vi "GVSGet Boolean Reference.vi"(8 "Label Name":string, 11 "VI Refnum":refnum<vi>) -> (1 "Boolean":bool, 2 "Boolean Ref":refnum<vi>, 3 "VI Refnum Out":refnum<vi>)   [LabVIEW 2013]
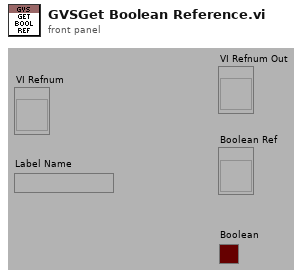
[diagram p1: front panel]
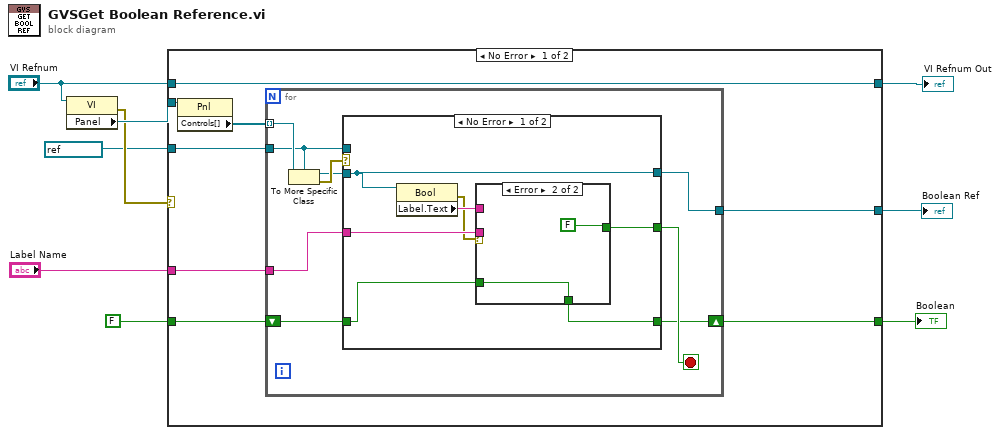
[diagram p0: block diagram]
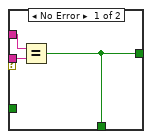
[diagram p2: hidden frame]
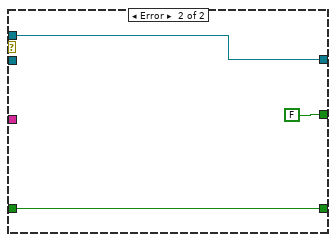
[diagram p3: hidden frame]
diagram:
  n1 = property class="VI"(reference="VI Refnum") -> (error out=w6:errorcluster, "Panel"=w8:refnum<vi>)  [unwired: 1 in, 1 out]
  n2 = case shown="No Error" w6 {
    tunnel: "Label Name" -> [w17 _]
    tunnel: w8 -> [w16 _]
    tunnel: "VI Refnum" -> [w11 w44]
    tunnel: FALSE ("Boolean") -> [w14 w42]
    tunnel: [w13 w42] -> w4
    tunnel: [w12 w43] -> w3
    tunnel: [w11 w44] -> w2
    tunnel: refnum<vi> refnum ("Boolean") -> [w10 w43]
    frame No Error {
      n3 = property class="Pnl"(reference=w16) -> ("Controls[]"=w15:refnum<vi>[])  [unwired: 1 in, 2 out]
      n4 = for {
        tunnel: w15 -> [w26] mode=indexing
        tunnel: [w22] -> w12
        tunnel: w17 -> [w21]
        tunnel: w10 -> [w20]
        shift-right: [w18] -> w13
        shift-left: w14 -> [w19]
        stop <- w23 stop-if-true
        n5 = To More Specific Class(target class=w20, reference=w26) -> (specific class reference=w24:refnum<vi>, error out=w25:errorcluster)  [unwired: 1 in]
        n6 = case shown="No Error" w25 {
          tunnel: w24 -> [w31 _]
          tunnel: [w29 FALSE] -> w23
          tunnel: [w31 w40] -> w22
          tunnel: w21 -> [w32 _]
          tunnel: w20 -> [_ w40]
          tunnel: [w28 w39] -> w18
          tunnel: w19 -> [w27 w39]
          frame No Error {
            n7 = property class="Bool"(reference=w31) -> (error out=w30:errorcluster, "Label.Text"=w33:string)  [unwired: 1 in, 1 out]
            n8 = case shown="Error" w30 {
              tunnel: w33 -> [w36 _]
              tunnel: w32 -> [w35 _]
              tunnel: [w34 FALSE] -> w29
              tunnel: [w34 w37] -> w28
              tunnel: w27 -> [_ w37]
              frame No Error {
                n9 = Equal?(x=w36, y=w35) -> (x = y?=w34:bool)
              }
              frame Error {
              }
            }
          }
          frame Error {
          }
        }
      }
    }
    frame Error {
    }
  }
  "Boolean" <- w4
  "VI Refnum Out" <- w2
  "Boolean Ref" <- w3
